vi "Execute Function.vi"(8 "error in (no error)":errorcluster, 10 "Modbus request":refnum<class "Modbus Data Unit (PDU).lvclass">, 11 "device data model in":refnum<class "Device Data Model.lvclass">) -> (0 "error out":errorcluster, 2 "Modbus response":refnum<class "Modbus Data Unit (PDU).lvclass">, 3 "device data model out":refnum<class "Device Data Model.lvclass">)   [LabVIEW 2017, in "SubVIs.lvlib" / "Device Data Model.lvclass"]
doc: "This function is responsible for deciding what code to execute when a specific function is called."
uses:
  <vilib>/Modbus/subvis/Data and Functions/Device Data Model/Device Data Model.lvclass
  <vilib>/Modbus/subvis/Modbus Data Unit (PDU)/Modbus Data Unit (PDU).lvclass
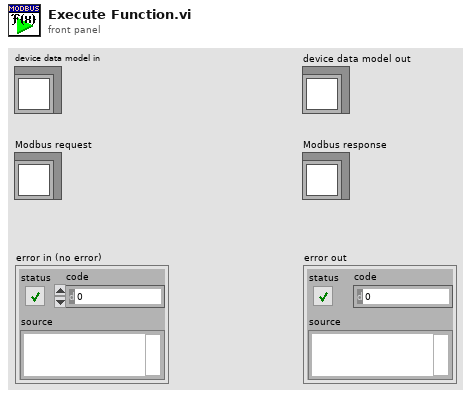
[diagram p1: front panel]
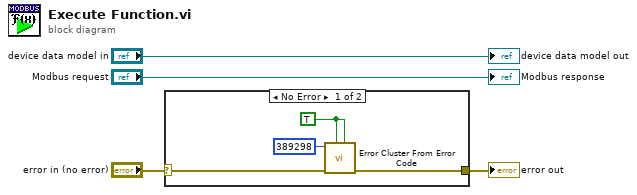
[diagram p0: block diagram]
diagram:
  n1 = case shown="No Error" "error in (no error)" {
    selector: "error in (no error)" -> [w8 w9]
    tunnel: [w7 w9] -> w1
    frame No Error {
      w5 = TRUE ("show call chain? (False)")
      n2 = call <vilib>:"Error Cluster From Error Code.vi"("is warning? (False)"=w5, "show call chain? (False)"=w5, "error in (no error)"=w8, "error code (0)"=389298) -> ("error out"=w7:errorcluster)  [unwired: 5 in]
    }
    frame Error {
    }
  }
  "error out" <- w1
  "device data model out" <- "device data model in"
  "Modbus response" <- "Modbus request"
